vi "Post-Build Action.vi"(5 "Files Generated by Build":path[](array[path]), 6 "Top Level/Always Included VIs":path[](array[path]), 7 "Destination Path":path, 8 "error in (no error)":errorcluster, 9 "Target Name":string, 10 "Build Specification Name":string, 11 "Project Path":path) -> (0 "error out":errorcluster)   [LabVIEW 2016]
uses:
  <vilib>/Utility/sysdir.llb/System Directory Type.ctl
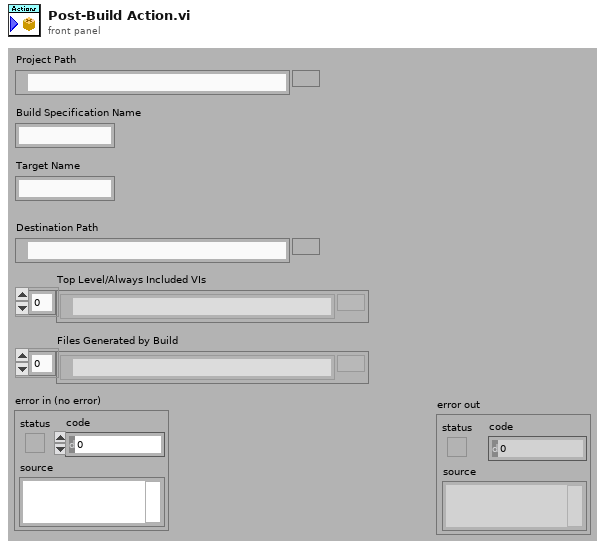
[diagram p1: front panel]
types:
  T1 = typedef "System Directory Type.ctl" = i32
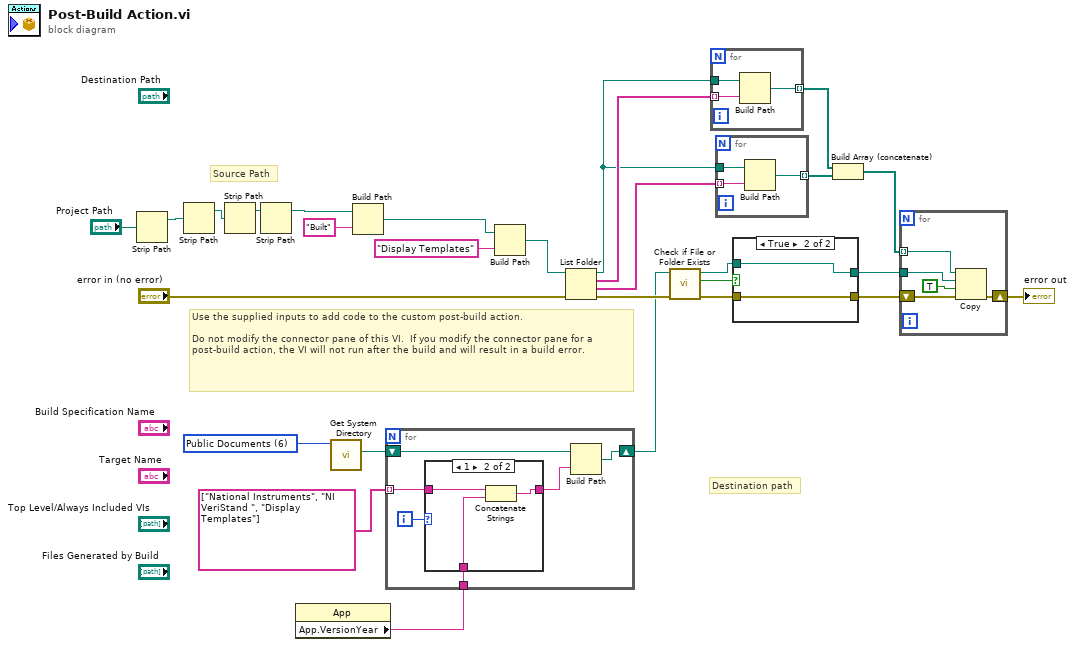
[diagram p0: block diagram]
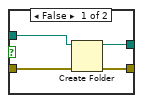
[diagram p3: hidden frame]
diagram:
  w10 = T1 6 items=["User Home"=0, "User Desktop"=1, "User Documents"=2, "User Application Data"=3, "User Preferences"=4, "User Temporary"=5, "Public Documents"=6, "Public Application Data"=7, "Public Preferences"=8, "Public Cache"=13, "System Core Libraries"=9, "System Installed Libraries"=10, "Application Files"=11, "Boot Volume Root"=12] ("system directory type")
  # "Destination path"
  # "Source Path"
  # "Use the supplied inputs to add code to the custom post-build action.\n\nDo not modify the connector pane of this VI.  If you modify the connector pane for a post-build action, the VI will not run after the build and will result in a build error."
  n1 = Strip Path(path="Project Path") -> (stripped path=w14:path)  [unwired: 1 out]
  n2 = Strip Path(path=w14) -> (stripped path=w3:path)  [unwired: 1 out]
  n3 = Strip Path(path=w3) -> (stripped path=w2:path)  [unwired: 1 out]
  n4 = Strip Path(path=w2) -> (stripped path=w1:path)  [unwired: 1 out]
  n5 = property class="App"() -> ("App.VersionYear"=w6:string)  [unwired: 2 in, 2 out]
  n6 = call <vilib>:"Get System Directory.vi"("system directory type"=w10) -> ("system directory"=w9:path)  [unwired: 10 in]
  n7 = Build Path(base path=w1, name or relative path="Built") -> (appended path=w5:path)
  n8 = for {
    shift-right: [w33] -> w7
    shift-left: w9 -> [w34]
    tunnel: string[] ["National Instruments", "NI VeriStand ", "Display Templates"] -> [w30] mode=indexing
    tunnel: w6 -> [w29]
    i -> [w32]
    n9 = case shown="1" w32 {
      tunnel: [w35 w37] -> w31
      tunnel: w30 -> [w35 w38]
      tunnel: w29 -> [_ w36]
      frame Default {
      }
      frame 1 {
        n10 = Concatenate Strings(w38, w36) -> (w37:string)
      }
    }
    n11 = Build Path(base path=w34, name or relative path=w31) -> (appended path=w33:path)
  }
  n12 = Build Path(base path=w5, name or relative path="Display Templates") -> (appended path=w13:path)
  n13 = List Folder(path=w13, error in="error in (no error)") -> (path out=w16:path, filenames=w28:string[], folder names=w17:string[], error out=w11:errorcluster)  [unwired: 2 in]
  n14 = call <vilib>:"Check if File or Folder Exists.vi"("error in (no error)"=w11, "path"=w7) -> ("error out"=w20:errorcluster, "file or folder exists?"=w22:bool, "dup path"=w21:path)  [unwired: 7 in]
  n15 = for {
    tunnel: w28 -> [w40] mode=indexing
    tunnel: w16 -> [w41]
    tunnel: [w39] -> w27 mode=indexing
    n16 = Build Path(base path=w41, name or relative path=w40) -> (appended path=w39:path)
  }
  n17 = for {
    tunnel: w17 -> [w43] mode=indexing
    tunnel: w16 -> [w44]
    tunnel: [w42] -> w15 mode=indexing
    n18 = Build Path(base path=w44, name or relative path=w43) -> (appended path=w42:path)
  }
  n19 = case shown="True" w22 {
    tunnel: w21 -> [w48 w50]
    tunnel: w20 -> [w47 w49]
    tunnel: [w46 w50] -> w19
    tunnel: [w45 w49] -> w18
    frame False {
      n20 = Create Folder(path (use dialog)=w48, error in=w47) -> (created path=w46:path, error out=w45:errorcluster)  [unwired: 1 in, 1 out]
    }
    frame True {
    }
  }
  n21 = Build Array (concatenate)(w27, w15) -> (w26:path[])
  n22 = for {
    tunnel: w26 -> [w52] mode=indexing
    shift-right: [w53] -> w4
    shift-left: w18 -> [w54]
    tunnel: w19 -> [w51]
    n23 = Copy(8:w54, 9:TRUE ("overwrite (F)"), 10:w51, 11:w52) -> (0:w53:errorcluster)  [unwired: 1 in, 2 out]
  }
  "error out" <- w4
